vi "Color Shift.vi"(1 "Color":T1(ring)) -> (0 "Color Box":u32(colorbox))   [LabVIEW 2017]
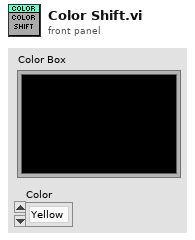
[diagram p1: front panel]
types:
  T1 = enum16{"Yellow", "Purple", "Green", "Blue", "Red"}
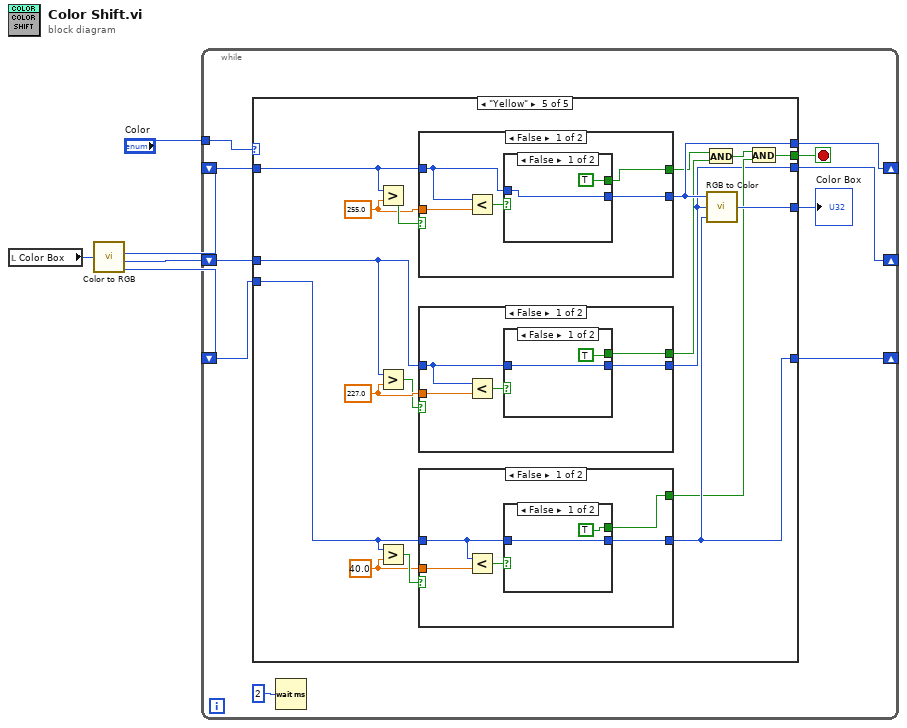
[diagram p0: block diagram]
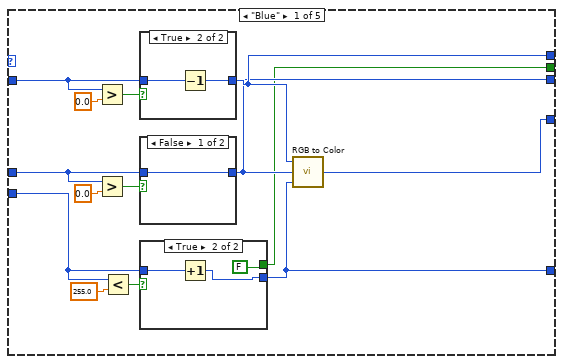
[diagram p2: hidden frame]
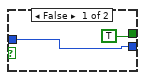
[diagram p3: hidden frame]
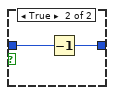
[diagram p4: hidden frame]
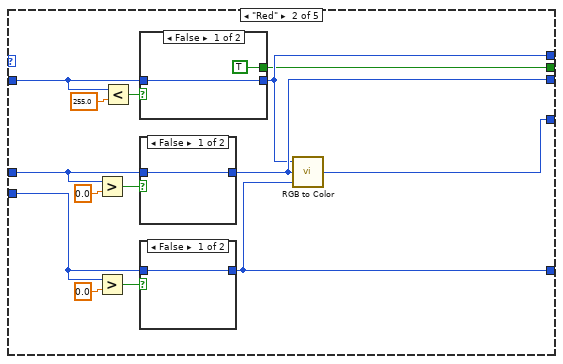
[diagram p6: hidden frame]
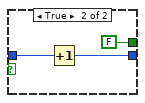
[diagram p7: hidden frame]
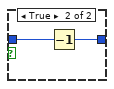
[diagram p8: hidden frame]
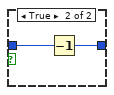
[diagram p9: hidden frame]
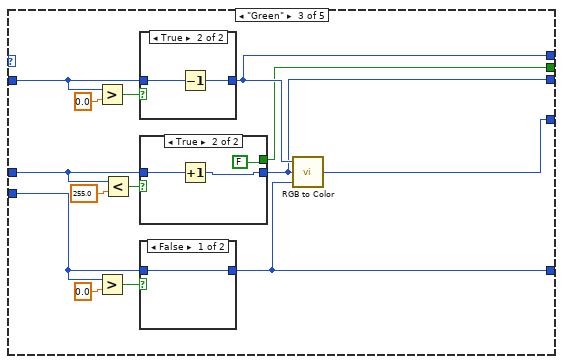
[diagram p10: hidden frame]
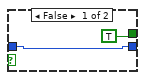
[diagram p11: hidden frame]
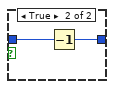
[diagram p13: hidden frame]
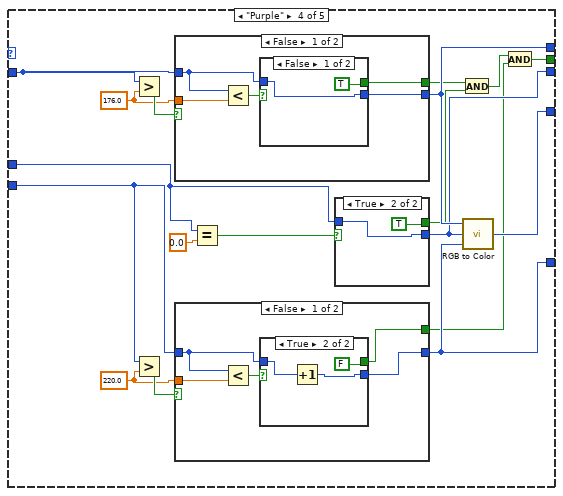
[diagram p14: hidden frame]
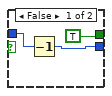
[diagram p15: hidden frame]
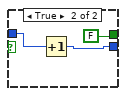
[diagram p16: hidden frame]
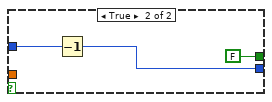
[diagram p17: hidden frame]
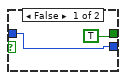
[diagram p18: hidden frame]
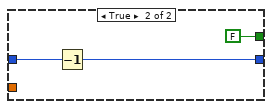
[diagram p19: hidden frame]
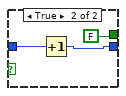
[diagram p20: hidden frame]
diagram:
  n1 = local read "Color Box"() -> (w5:u32)
  n2 = call <vilib>:"Color to RGB.vi"("Color"=w5) -> ("R"=w4:u8, "G"=w3:u8, "B"=w2:u8)  [unwired: 1 out]
  n3 = while {
    shift-right: [w11] -> _
    shift-left: w4 -> [w15]
    shift-right: [w10] -> _
    shift-left: w3 -> [w14]
    shift-right: [w9] -> _
    shift-left: w2 -> [w13]
    tunnel: "Color" -> [w6]
    stop <- w8 stop-if-true
    n4 = case shown="\"Yellow\"" w6 {
      tunnel: [w29 w48 w68 w99 w151] -> w11
      tunnel: w15 -> [w28 w49 w76 w105 w154]
      tunnel: w14 -> [w27 w54 w75 w104 w142]
      tunnel: w13 -> [w26 w51 w78 w107 w156]
      tunnel: [w25 w53 w67 w98 w140] -> w10
      tunnel: [w24 w50 w77 w106 w155] -> w9
      tunnel: [w23 w52 w79 w108 w157] -> w12
      tunnel: [w16 w41 w66 w91 w145] -> w8
      frame "Blue" {
        n5 = Greater?(x=w28, y=0.0) -> (0:w21:bool)
        n6 = Greater?(x=w27, y=0.0) -> (0:w20:bool)
        n7 = Less?(x=w26, y=255.0) -> (x < y?=w18:bool)
        n8 = case shown="True" w21 {
          tunnel: [w38 w40] -> w29
          tunnel: w28 -> [w38 w39]
          frame False {
          }
          frame True {
            n9 = Decrement(x=w39) -> (x-1=w40:u8)
          }
        }
        n10 = case shown="False" w20 {
          tunnel: [w35 w37] -> w25
          tunnel: w27 -> [w35 w36]
          frame False {
          }
          frame True {
            n11 = Decrement(x=w36) -> (x-1=w37:u8)
          }
        }
        n12 = case shown="True" w18 {
          tunnel: [w31 w34] -> w24
          tunnel: w26 -> [w31 w33]
          tunnel: [TRUE FALSE] -> w16
          frame False {
          }
          frame True {
            n13 = Increment(x=w33) -> (x+1=w34:u8)
          }
        }
        n14 = call <vilib>:"RGB to Color.vi"("B"=w24, "G"=w25, "R"=w29) -> ("Color"=w23:u32)
      }
      frame "Red" {
        n15 = Greater?(x=w54, y=0.0) -> (0:w47:bool)
        n16 = Greater?(x=w51, y=0.0) -> (0:w45:bool)
        n17 = Less?(x=w49, y=255.0) -> (x < y?=w43:bool)
        n18 = case shown="False" w43 {
          tunnel: [w56 w59] -> w48
          tunnel: w49 -> [w56 w58]
          tunnel: [TRUE FALSE] -> w41
          frame False {
          }
          frame True {
            n19 = Increment(x=w58) -> (x+1=w59:u8)
          }
        }
        n20 = case shown="False" w47 {
          tunnel: [w63 w65] -> w53
          tunnel: w54 -> [w63 w64]
          frame False {
          }
          frame True {
            n21 = Decrement(x=w64) -> (x-1=w65:u8)
          }
        }
        n22 = case shown="False" w45 {
          tunnel: [w60 w62] -> w50
          tunnel: w51 -> [w60 w61]
          frame False {
          }
          frame True {
            n23 = Decrement(x=w61) -> (x-1=w62:u8)
          }
        }
        n24 = call <vilib>:"RGB to Color.vi"("B"=w50, "G"=w53, "R"=w48) -> ("Color"=w52:u32)
      }
      frame "Green" {
        n25 = Greater?(x=w76, y=0.0) -> (0:w71:bool)
        n26 = Greater?(x=w78, y=0.0) -> (0:w74:bool)
        n27 = Less?(x=w75, y=255.0) -> (x < y?=w70:bool)
        n28 = case shown="True" w71 {
          tunnel: [w85 w87] -> w68
          tunnel: w76 -> [w85 w86]
          frame False {
          }
          frame True {
            n29 = Decrement(x=w86) -> (x-1=w87:u8)
          }
        }
        n30 = case shown="True" w70 {
          tunnel: [w81 w84] -> w67
          tunnel: w75 -> [w81 w83]
          tunnel: [TRUE FALSE] -> w66
          frame False {
          }
          frame True {
            n31 = Increment(x=w83) -> (x+1=w84:u8)
          }
        }
        n32 = case shown="False" w74 {
          tunnel: [w88 w90] -> w77
          tunnel: w78 -> [w88 w89]
          frame False {
          }
          frame True {
            n33 = Decrement(x=w89) -> (x-1=w90:u8)
          }
        }
        n34 = call <vilib>:"RGB to Color.vi"("B"=w77, "G"=w67, "R"=w68) -> ("Color"=w79:u32)
      }
      frame "Purple" {
        w97 = 176.0 ("y")
        w96 = 220.0 ("y")
        n35 = Greater?(x=w105, y=w97) -> (0:w102:bool)
        n36 = Greater?(x=w107, y=w96) -> (0:w103:bool)
        n37 = case shown="False" w102 {
          tunnel: [w115 w126] -> w99
          tunnel: w105 -> [w116 w125]
          tunnel: w97 -> [w118 _]
          tunnel: [w114 FALSE] -> w95
          frame False {
            n38 = Less?(x=w116, y=w118) -> (x < y?=w117:bool)
            n39 = case shown="False" w117 {
              tunnel: w116 -> [w120 w123]
              tunnel: [w120 w122] -> w115
              tunnel: [TRUE FALSE] -> w114
              frame False {
              }
              frame True {
                n40 = Increment(x=w123) -> (x+1=w122:u8)
              }
            }
          }
          frame True {
            n41 = Decrement(x=w125) -> (x-1=w126:u8)
          }
        }
        n42 = case shown="False" w103 {
          tunnel: [w128 w139] -> w106
          tunnel: w107 -> [w129 w138]
          tunnel: w96 -> [w131 _]
          tunnel: [w127 FALSE] -> w93
          frame False {
            n43 = Less?(x=w129, y=w131) -> (x < y?=w130:bool)
            n44 = case shown="True" w130 {
              tunnel: w129 -> [w133 w136]
              tunnel: [w133 w135] -> w128
              tunnel: [TRUE FALSE] -> w127
              frame False {
              }
              frame True {
                n45 = Increment(x=w136) -> (x+1=w135:u8)
              }
            }
          }
          frame True {
            n46 = Decrement(x=w138) -> (x-1=w139:u8)
          }
        }
        n47 = Equal?(x=w104, y=0.0) -> (x = y?=w101:bool)
        n48 = case shown="True" w101 {
          tunnel: [w109 w112] -> w98
          tunnel: w104 -> [w110 w112]
          tunnel: [TRUE TRUE] -> w94
          frame False {
            n49 = Decrement(x=w110) -> (x-1=w109:u8)
          }
          frame True {
          }
        }
        n50 = And(x=w95, y=w94) -> (x .and. y?=w92:bool)
        n51 = call <vilib>:"RGB to Color.vi"("B"=w106, "G"=w98, "R"=w99) -> ("Color"=w108:u32)
        n52 = And(x=w92, y=w93) -> (x .and. y?=w91:bool)
      }
      frame "Yellow" {
        w144 = 227.0 ("y")
        w150 = 255.0 ("y")
        w149 = 40.0 ("y")
        n53 = Greater?(x=w154, y=w150) -> (0:w152:bool)
        n54 = Greater?(x=w142, y=w144) -> (0:w143:bool)
        n55 = Greater?(x=w156, y=w149) -> (0:w153:bool)
        n56 = case shown="False" w152 {
          tunnel: [w172 w183] -> w151
          tunnel: w154 -> [w173 w182]
          tunnel: w150 -> [w175 _]
          tunnel: [w171 FALSE] -> w148
          frame False {
            n57 = Less?(x=w173, y=w175) -> (x < y?=w174:bool)
            n58 = case shown="False" w174 {
              tunnel: w173 -> [w177 w180]
              tunnel: [w177 w179] -> w172
              tunnel: [TRUE FALSE] -> w171
              frame False {
              }
              frame True {
                n59 = Increment(x=w180) -> (x+1=w179:u8)
              }
            }
          }
          frame True {
            n60 = Decrement(x=w182) -> (x-1=w183:u8)
          }
        }
        n61 = case shown="False" w143 {
          tunnel: [w159 w170] -> w140
          tunnel: w142 -> [w160 w169]
          tunnel: w144 -> [w162 _]
          tunnel: [w158 FALSE] -> w141
          frame False {
            n62 = Less?(x=w160, y=w162) -> (x < y?=w161:bool)
            n63 = case shown="False" w161 {
              tunnel: w160 -> [w164 w167]
              tunnel: [w164 w166] -> w159
              tunnel: [TRUE FALSE] -> w158
              frame False {
              }
              frame True {
                n64 = Increment(x=w167) -> (x+1=w166:u8)
              }
            }
          }
          frame True {
            n65 = Decrement(x=w169) -> (x-1=w170:u8)
          }
        }
        n66 = case shown="False" w153 {
          tunnel: [w185 w196] -> w155
          tunnel: w156 -> [w186 w195]
          tunnel: w149 -> [w188 _]
          tunnel: [w184 FALSE] -> w147
          frame False {
            n67 = Less?(x=w186, y=w188) -> (x < y?=w187:bool)
            n68 = case shown="False" w187 {
              tunnel: w186 -> [w190 w193]
              tunnel: [w190 w192] -> w185
              tunnel: [TRUE FALSE] -> w184
              frame False {
              }
              frame True {
                n69 = Increment(x=w193) -> (x+1=w192:u8)
              }
            }
          }
          frame True {
            n70 = Decrement(x=w195) -> (x-1=w196:u8)
          }
        }
        n71 = And(x=w148, y=w141) -> (x .and. y?=w146:bool)
        n72 = call <vilib>:"RGB to Color.vi"("B"=w155, "G"=w140, "R"=w151) -> ("Color"=w157:u32)
        n73 = And(x=w146, y=w147) -> (x .and. y?=w145:bool)
      }
    }
    "Color Box" <- w12
    n74 = Wait (ms)(milliseconds to wait=u32 2) -> ()  [unwired: 1 out]
  }
